vi "Detect.vi"(0 "Interface":string, 1 "USB (True)":bool=TRUE, 2 "Wi-Fi within local segment (False)":bool, 3 "Wi-Fi specified IPv4 address  (False)":bool, 5 "DeviceName":string="GFX100", 11 "error in (no error)":errorcluster) -> (4 "Result":i32, 6 "Count":i32, 15 "error out":errorcluster)   [LabVIEW 2018, in "Fujifilm X Series GFX System Digital Camera.lvlib"]
doc: "Enumerates available cameras and generate a connected camera list."
uses:
  <instrlib>/Fujifilm X Series GFX System Digital Camera/Fujifilm X Series GFX System Digital Camera.lvlib
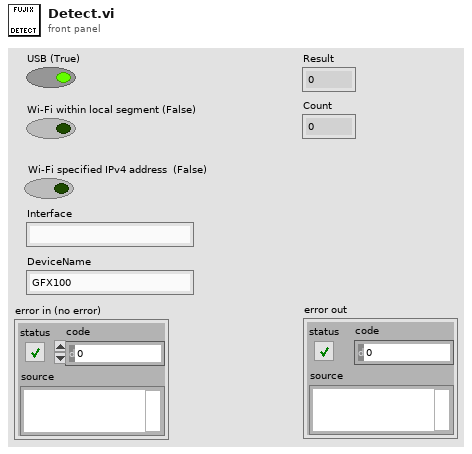
[diagram p1: front panel]
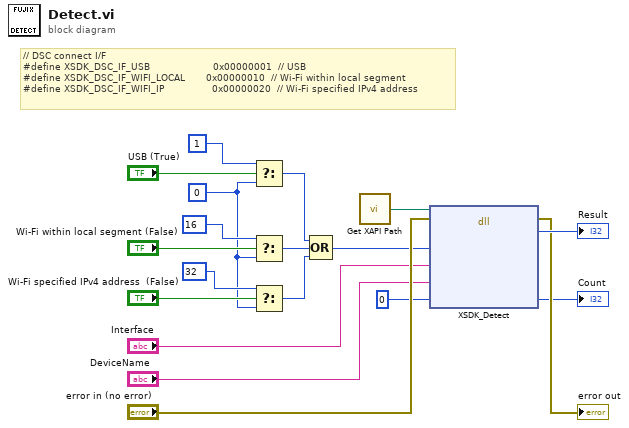
[diagram p0: block diagram]
diagram:
  w6 = 0
  # "// DSC connect I/F\n#define XSDK_DSC_IF_USB                     0x00000001  // USB\n#define XSDK_DSC_IF_WIFI_LOCAL       0x00000010  // Wi-Fi within local segment\n#define XSDK_DSC_IF_WIFI_IP                0x00000020  // Wi-Fi specified IPv4 address"
  n1 = Select(t=1, s="USB (True)", f=w6) -> (s? t:f=w9:i32)
  n2 = Select(t=16, s="Wi-Fi within local segment (False)", f=w6) -> (s? t:f=w8:i32)
  n3 = Select(t=32, s="Wi-Fi specified IPv4 address  (False)", f=w6) -> (s? t:f=w7:i32)
  n4 = Compound Arithmetic op=OR(w9, w8, w7) -> (w5:i32)
  n5 = call <instrlib>:"Get XAPI Path.vi"() -> ("XAPI Library Path"=w19:path)  [unwired: 1 in]
  n6 = dll-call lib="E:/fuji/SDK13100/REDISTRIBUTABLES/Windows/32bit/XAPI.dll" fn="XSDK_Detect"(path in=w19, error in="error in (no error)", "lInterface"=w5, "pInterface"="Interface", "pDeviceName"="DeviceName", "plCount"=0) -> (error out=→"error out":errorcluster, "result"=→"Result":i32, "plCount"=→"Count":i32)  [unwired: 4 in, 1 out]
